vi "upload_file.vi"(8 "error in (no error)":errorcluster, 9 "portal_upload_path":string="https://siasky.net/", 10 "portal_url":string="https://siasky.net/", 11 "Local File Path":path=path "D:/") -> (0 "error out":errorcluster)   [LabVIEW 2019, in "SiaSkynetAPI.lvlib"]
uses:
  SiaSkynetAPI.lvlib
  <vilib>/httpClient/MultipartData.ctl
  <vilib>/httpClient/LabVIEWHTTPClient.lvlib
panel:
  out "skylink":string
  out "body":string
  out "headers":string
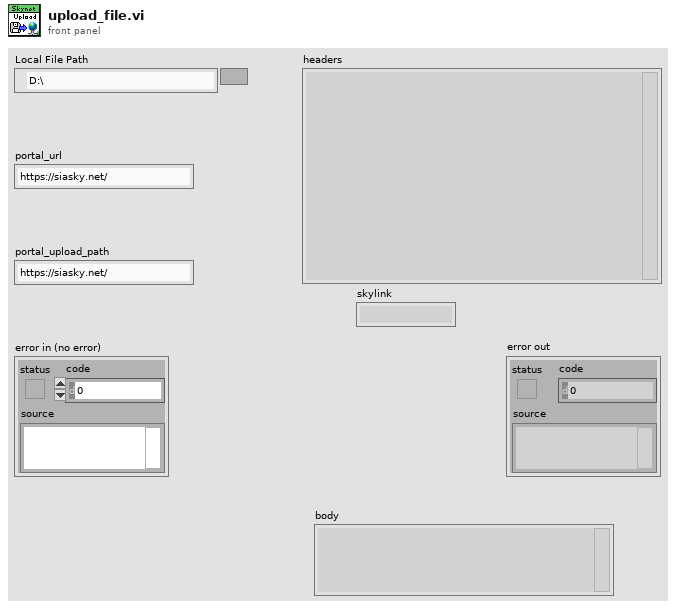
[diagram p1: front panel]
types:
  T1 = typedef "LabVIEWHTTPClient.lvlib/MultipartData.ctl" = cluster{"Name":string, "Value":string, "File":path, "Filename":string, "MIME type":string}
  T2 = typedef "LabVIEWHTTPClient.lvlib/ClientHandle.ctl" = refnum<k1>
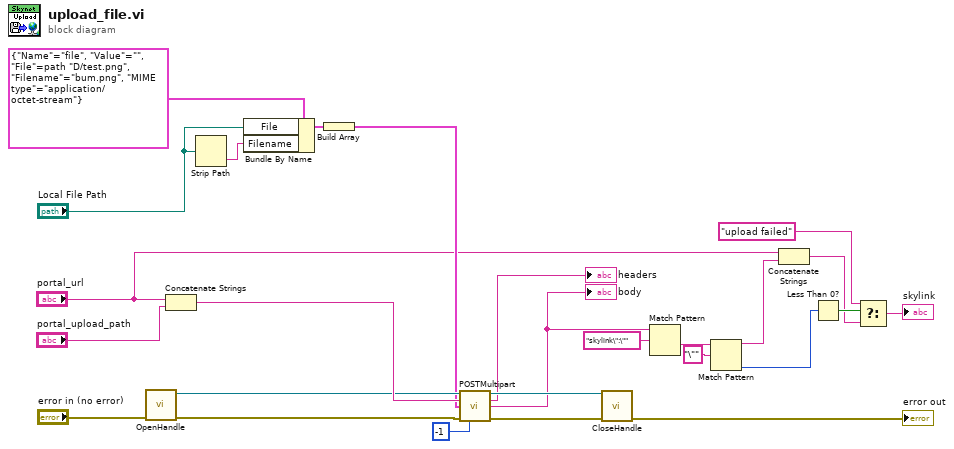
[diagram p0: block diagram]
diagram:
  n1 = call <vilib>:"OpenHandle.vi"("error in (no error)"="error in (no error)") -> ("client handle out"=w20:T2, "error out"=w19:errorcluster)  [unwired: 13 in]
  n2 = Concatenate Strings("portal_url", "portal_upload_path") -> (w21:string)
  n3 = Strip Path(path="Local File Path") -> (name=w12:string)  [unwired: 1 out]
  n4 = Bundle By Name(cluster=T1 {"Name"="file", "Value"="", "File"=path "D:/test.png", "Filename"="bum.png", "MIME type"="application/octet-stream"} ("Element"), "File"="Local File Path", "Filename"=w12) -> (w15:T1)
  n5 = Build Array(w15) -> (w14:T1[])
  n6 = call <vilib>:"POSTMultipart.vi"("client handle"=w20, "url"=w21, "data"=w14, "error in (no error)"=w19, "timeout (10000)"=-1) -> ("client handle out"=w26:T2, "headers"=→"headers":string, "body"=w11:string, "error out"=w25:errorcluster)  [unwired: 7 in]
  "body" <- w11
  n7 = call <vilib>:"CloseHandle.vi"("client handle"=w26, "error in (no error)"=w25) -> ("error out"=→"error out":errorcluster)  [unwired: 13 in]
  n8 = Match Pattern(string=w11, regular expression="skylink\":\"") -> (after substring=w9:string)  [unwired: 1 in, 3 out]
  n9 = Match Pattern(string=w9, regular expression="\"") -> (before substring=w6:string, offset past match=w4:i32)  [unwired: 1 in, 2 out]
  n10 = Concatenate Strings("portal_url", w6) -> (w3:string)
  n11 = Less Than 0?(x=w4) -> (x < 0?=w5:bool)
  n12 = Select(t="upload failed", s=w5, f=w3) -> (s? t:f=→"skylink":string)
